vi "TIO Stream Read.vi"(8 "error in (no error)":errorcluster, 11 "TS Connection":T2={"Type"=enum."TCP", "Serial"="serial:///dev/cu.usbserial-00000", "TCP"=refnum, "Timeout"=500}) -> (0 "error out":errorcluster, 1 "Payload":string, 2 "Type":T1(ring)=enum."RPC Request", 3 "TS Connection":T2={"Type"=enum."TCP", "Serial"="serial:///dev/cu.usbserial-00000", "TCP"=refnum, "Timeout"=500})   [LabVIEW 2017]
uses:
  Helpers/TIO Serial Checksum CRC32.vi
panel:
  out "Routing Size":u8
  out "Payload Length":u16
  # "TODO Handle routing"
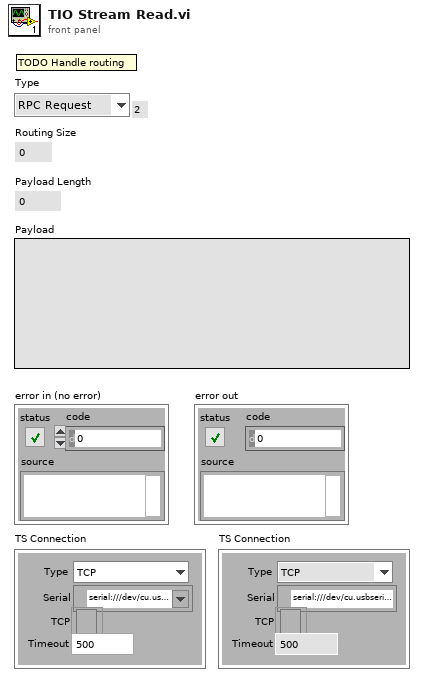
[diagram p1: front panel]
types:
  T1 = enum8{"Invalid", "Log", "RPC Request", "RPC Reply", "RPC Error", "Stream Description", "User"}
  T2 = cluster{"Type":enum16{"TCP", "Serial"}, "Serial":refnum<visa-resource-name>, "TCP":refnum<k5>, "Timeout":u32}
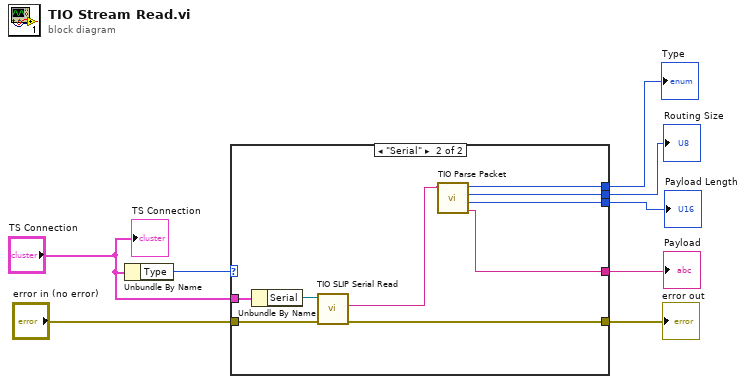
[diagram p0: block diagram]
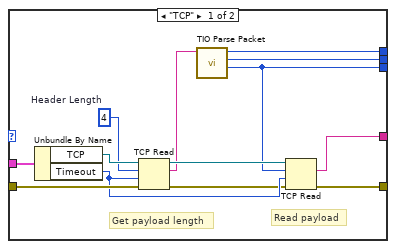
[diagram p2: hidden frame]
diagram:
  n1 = Unbundle By Name("TS Connection") -> ("Type"=w6:enum16{"TCP", "Serial"})
  n2 = case shown="\"Serial\"" w6 {
    tunnel: "error in (no error)" -> [w18 w29]
    tunnel: [w17 w30] -> w8
    tunnel: "TS Connection" -> [w21 w28]
    tunnel: [w16 w23] -> w1
    tunnel: [w10 w24] -> w4
    tunnel: [w12 w25] -> w3
    tunnel: [w11 w26] -> w2
    frame "TCP" {
      w14 = u32 4  # Header Length
      # "Read payload"
      # "Get payload length"
      n3 = Unbundle By Name(w21) -> ("TCP"=w20:refnum<k5>, "Timeout"=w15:u32)
      n4 = TCP Read(connection ID=w20, bytes to read=w14, error in (no error)=w18, 9:w15) -> (connection ID out=w19:refnum<k5>, data out=w13:string, error out=w9:errorcluster)  [unwired: 1 in]
      n5 = call "TIO Parse Packet.vi"("Packet"=w13) -> ("Payload Length"=w10:u16, "Routing Size"=w12:u8, "Type"=w11:u16)  [unwired: 7 in, 1 out]
      n6 = TCP Read(connection ID=w19, bytes to read=w10, error in (no error)=w9, 9:w15) -> (data out=w16:string, error out=w17:errorcluster)  [unwired: 1 in, 1 out]
    }
    frame "Serial" {
      n7 = Unbundle By Name(w28) -> ("Serial"=w27:refnum<visa-resource-name>)
      n8 = call "TIO SLIP Serial Read.vi"("error in (no error)"=w29, "VISA resource name"=w27) -> ("error out"=w30:errorcluster, "Payload"=w22:string)  [unwired: 7 in, 1 out]
      n9 = call "TIO Parse Packet.vi"("Packet"=w22) -> ("Payload"=w23:string, "Payload Length"=w24:u16, "Routing Size"=w25:u8, "Type"=w26:u16)  [unwired: 7 in]
    }
  }
  "error out" <- w8
  "Payload" <- w1
  "Type" <- w2
  "Routing Size" <- w3
  "Payload Length" <- w4
  "TS Connection" <- "TS Connection"
